vi "DatabaseHandler_Core.vi"(0 "Object Refnum In":T3, 1 "Name":string, 2 "Object Data In":T2, 3 "subele index":i32, 4 "SubEle In":T1, 5 "error in (no error)":errorcluster, 6 "Function (Get Data)":T4=enum."Get Data") -> (11 "Valid Object":bool, 12 "Objects":T3[](array[typedef]), 13 "Created New":bool, 14 "Object Refnum out":T3, 15 "Name Out":string, 16 "Object Data Out":T2, 18 "object index":i32, 19 "error out":errorcluster)   [LabVIEW 2016]
doc: "This VI is the object core. It assigns a RefNum for each object as it is created using the Register function. Object data is accessed using the appropriate RefNum.\nCopyright 2001 VI Engineering, Inc."
uses:
  Database_Refnum.ctl
  DatabaseHand_Function.ctl
  DatabaseHand_Element.ctl
  DatabaseHan_DatabaseElement.ctl
  <vilib>/Utility/error.llb/whitespace.ctl
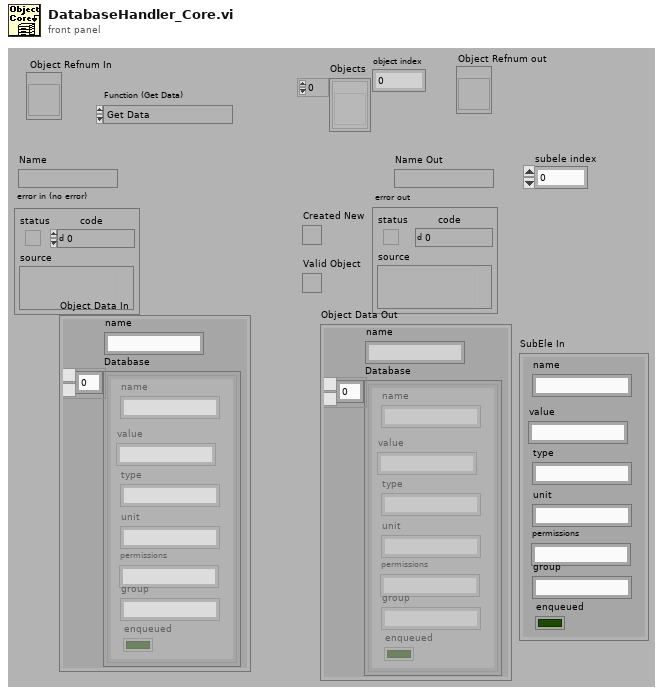
[diagram p1: front panel]
types:
  T1 = typedef "DatabaseHan_DatabaseElement.ctl" = cluster{"name":string, "value":string, "type":string, "unit":string, "permissions":string, "enqueued":bool, "group":string}
  T2 = typedef "DatabaseHand_Element.ctl" = cluster{"name":string, "Database":T1[]}
  T3 = typedef "Database_Refnum.ctl" = refnum<vi>
  T4 = typedef "DatabaseHand_Function.ctl" = enum16{"Reset", "Register", "Get Data", "Set Data", "Unregister", "Test", "Get Objects", "Delete Data"}
  T5 = typedef "whitespace.ctl" = u16
  T6 = typedef "Semaphore RefNum" = refnum<k1>
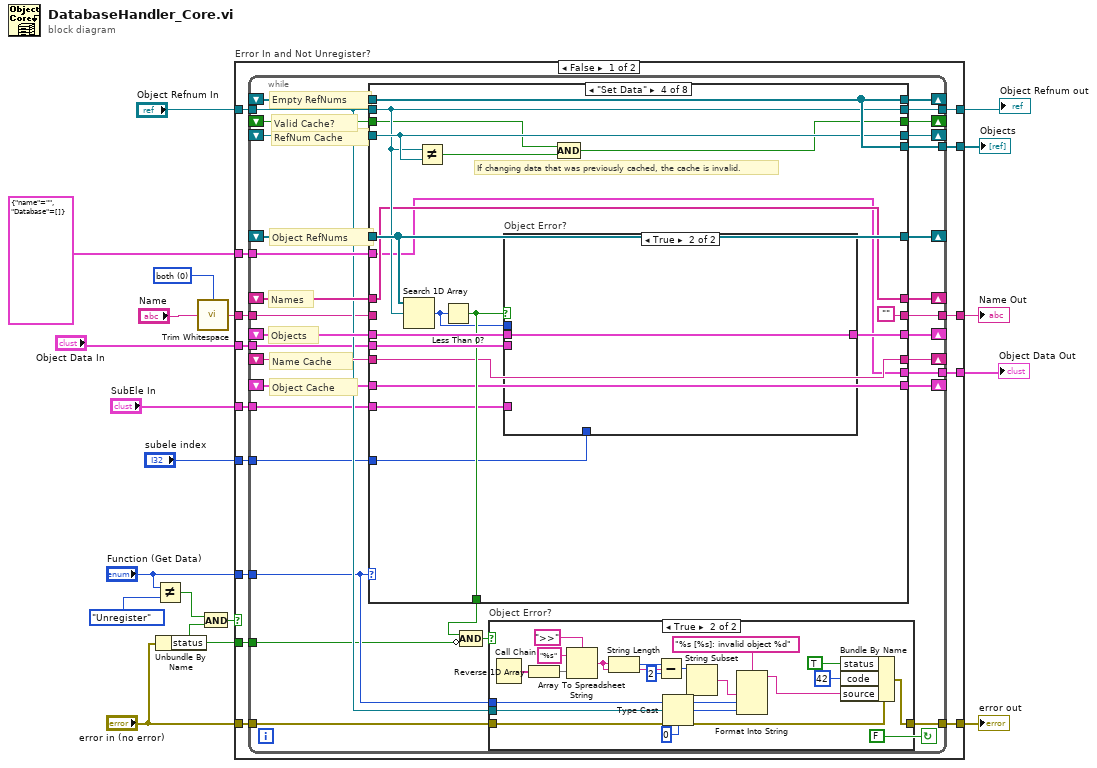
[diagram p0: block diagram]
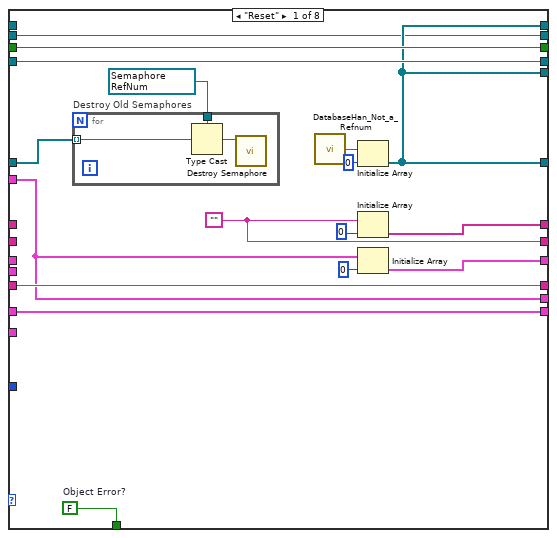
[diagram p3: hidden frame]
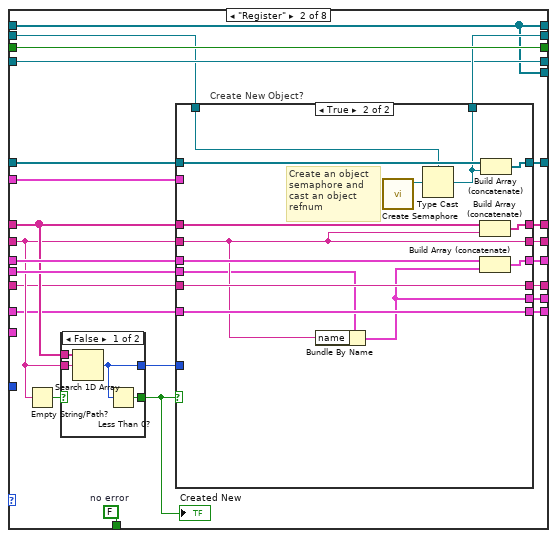
[diagram p4: hidden frame]
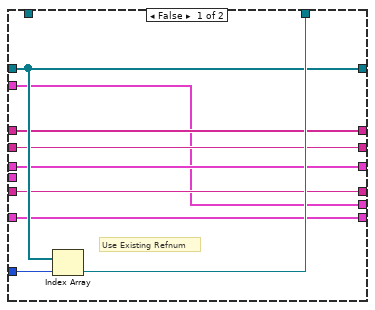
[diagram p5: hidden frame]
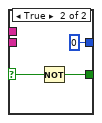
[diagram p6: hidden frame]
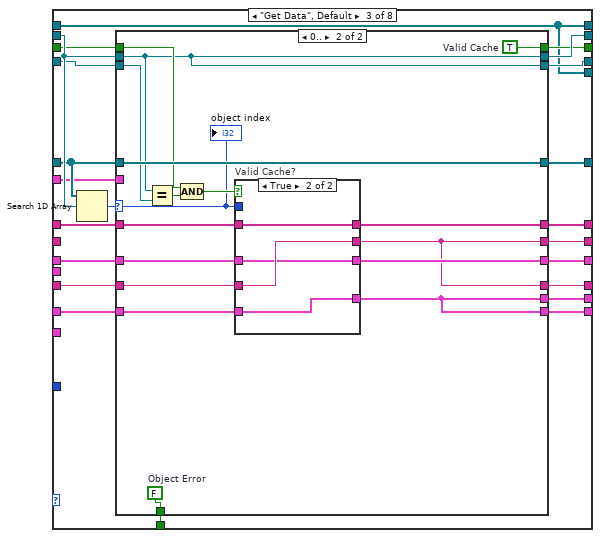
[diagram p7: hidden frame]
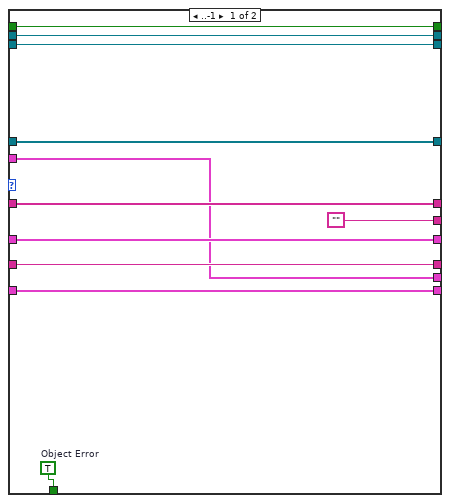
[diagram p8: hidden frame]
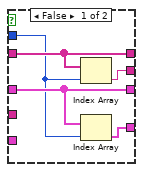
[diagram p9: hidden frame]
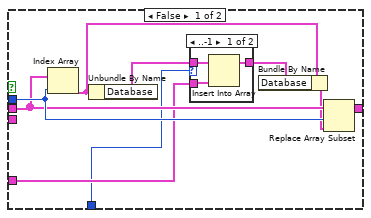
[diagram p10: hidden frame]
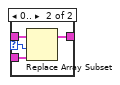
[diagram p11: hidden frame]
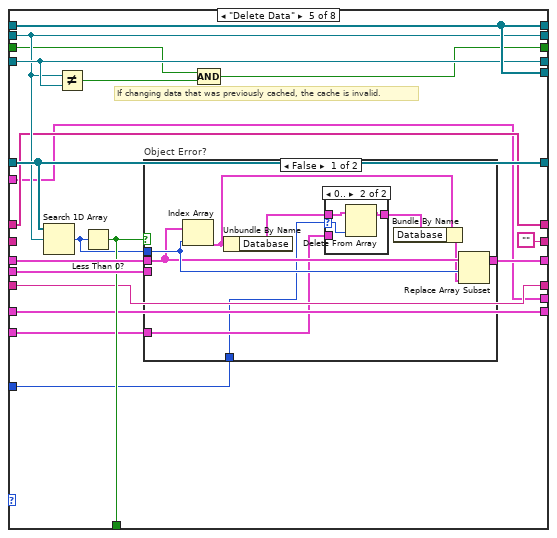
[diagram p12: hidden frame]
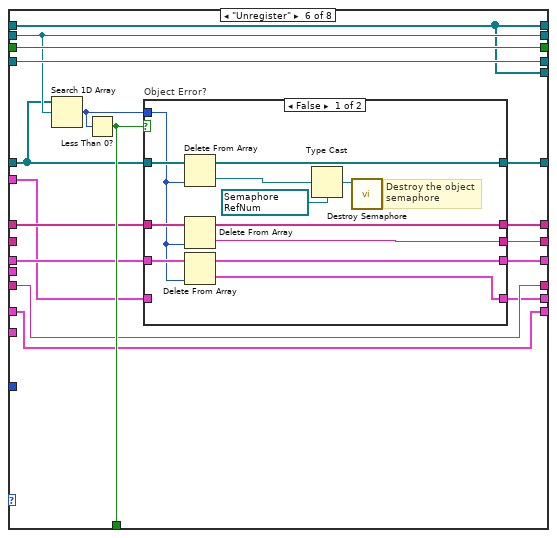
[diagram p15: hidden frame]
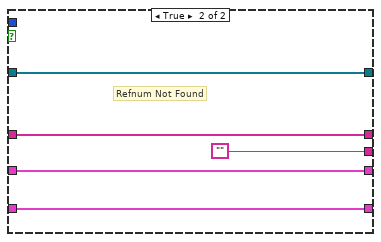
[diagram p16: hidden frame]
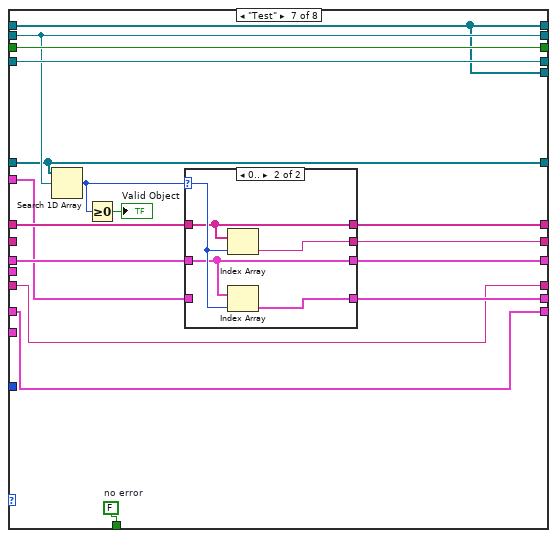
[diagram p17: hidden frame]
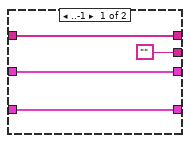
[diagram p18: hidden frame]
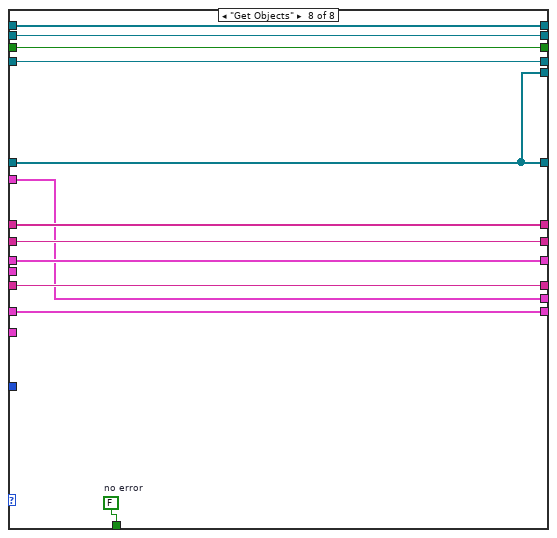
[diagram p19: hidden frame]
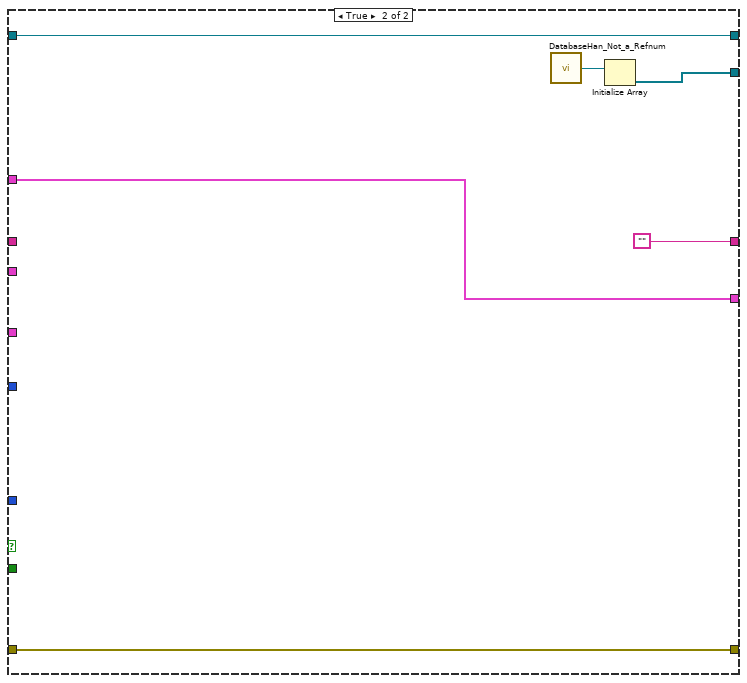
[diagram p20: hidden frame]
diagram:
  w1 = T5 0 items=["both", "start of string", "end of string"] ("location (both)")
  n1 = Not Equal?(x="Function (Get Data)", y=DatabaseHand_Function."Unregister") -> (x != y?=w13:bool)
  n2 = Unbundle By Name("error in (no error)") -> ("status"=w14:bool)
  n3 = call <vilib>:"Trim Whitespace.vi"("string"="Name", "location (both)"=w1) -> ("trimmed string"=w2:string)
  n4 = And(x=w13, y=w14) -> (x .and. y?=w12:bool)
  n5 = case "Error In and Not Unregister?" shown="False" w12 {
    tunnel: "Object Refnum In" -> [w33 w365]
    tunnel: cluster{"name":string, "Database":T1[]} {"name"="", "Database"=[]} ("Object Data In") -> [w32 w361]
    tunnel: "error in (no error)" -> [w31 w366]
    tunnel: [w30 w366] -> w19
    tunnel: "Object Data In" -> [w29 _]
    tunnel: [w28 w365] -> w10
    tunnel: w2 -> [w27 _]
    tunnel: [w26 ""] -> w17
    tunnel: [w25 w361] -> w8
    tunnel: [w24 w363] -> w6
    tunnel: "Function (Get Data)" -> [w23 _]
    tunnel: w14 -> [w22 _]
    tunnel: "SubEle In" -> [w21 _]
    tunnel: "subele index" -> [w20 _]
    frame False {
      n6 = while {
        tunnel: w22 -> [w39]
        shift-left: _ -> [w40]
        shift-right: [w41] -> _
        tunnel: [w42] -> w24
        tunnel: [w43] -> w25
        tunnel: [w44] -> w26
        tunnel: w27 -> [w45]
        tunnel: [w46] -> w28
        tunnel: w29 -> [w47]
        tunnel: [w48] -> w30
        tunnel: w31 -> [w51]
        shift-left: _ -> [w54]
        shift-right: [w53] -> _
        shift-left: _ -> [w56]
        shift-right: [w55] -> _
        shift-left: _ -> [w58]
        shift-right: [w57] -> _
        tunnel: w32 -> [w52]
        tunnel: w33 -> [w50]
        shift-left: _ -> [w60]
        shift-right: [w59] -> _
        shift-left: _ -> [w62]
        shift-right: [w61] -> _
        shift-left: _ -> [w64]
        shift-right: [w63] -> _
        shift-left: _ -> [w66]
        shift-right: [w65] -> _
        tunnel: w23 -> [w49]
        tunnel: w21 -> [w35]
        tunnel: w20 -> [w34]
        stop <- FALSE continue-if-true
        # "Empty RefNums"
        # "Object Cache"
        # "Name Cache"
        # "Names"
        # "Objects"
        # "Object RefNums"
        # "RefNum Cache"
        # "Valid Cache?"
        n7 = case shown="\"Set Data\"" w49 {
          tunnel: w50 -> [w91 w121 w181 w228 w264 w303 w337 w358]
          tunnel: w66 -> [w103 w130 w180 w225 w261 w304 w338 w359]
          tunnel: [w103 w130 w174 w227 w263 w304 w338 w359] -> w65
          tunnel: w64 -> [w102 w123 w179 w229 w265 w305 w339 w360]
          tunnel: [w102 w123 w173 w229 w265 w305 w339 w360] -> w63
          tunnel: w62 -> [w87 w122 w178 w231 w267 w301 w336 w349]
          tunnel: [w92 w129 w172 w231 w267 w298 w336 w349] -> w61
          tunnel: w60 -> [_ w128 w177 w237 w273 w299 w332 w352]
          tunnel: [w98 w127 w171 w236 w272 w295 w328 w352] -> w59
          tunnel: w58 -> [_ w120 w176 w226 w262 w300 w333 w354]
          tunnel: [w93 w124 w170 w226 w262 w296 w329 w354] -> w57
          tunnel: w56 -> [w101 w116 w169 w233 w269 w294 w325 w355]
          tunnel: [w101 w115 w165 w233 w269 w294 w325 w355] -> w55
          tunnel: w54 -> [w100 w114 w168 w232 w268 w293 w326 w356]
          tunnel: [w100 w113 w164 w232 w268 w293 w326 w356] -> w53
          tunnel: w52 -> [w89 w110 w162 w222 w258 w289 w327 w351]
          tunnel: [w95 w108 w163 w235 w271 w302 w335 w357] -> w37
          tunnel: w47 -> [_ w126 _ w238 w274 _ _ _]
          tunnel: [w91 w125 w175 w228 w264 w303 w337 w358] -> w46
          tunnel: w45 -> [_ w119 _ _ _ _ _ w353]
          tunnel: [w90 w112 w167 "" "" w291 w331 w353] -> w44
          tunnel: [w89 w111 w166 w222 w258 w290 w330 w351] -> w43
          tunnel: [w92 w109 w161 w230 w266 w292 w324 w349] -> w42
          tunnel: [w92 w109 w161 w230 w266 w292 w324 w350] -> w41
          tunnel: w40 -> [_ w109 w161 w230 w266 w292 w324 w350]
          tunnel: w35 -> [_ _ _ w221 w257 _ _ _]
          tunnel: w34 -> [_ _ _ w220 w256 _ _ _]
          frame "Reset" {
            w88 = T6 refnum items=["semaphore"] ("semaphore")
            w95 = FALSE  # Object Error?
            w90 = ""
            n8 = for "Destroy Old Semaphores" {
              tunnel: w87 -> [w105] mode=indexing
              tunnel: w88 -> [w106]
              n9 = Type Cast(type=w106, x=w105) -> (*(type *) &x=w104:T6)
              n10 = call <vilib>:"Destroy Semaphore.vi"("semaphore"=w104) -> ()  [unwired: 1 in, 6 out]
            }
            n11 = call "DatabaseHan_Not_a_Refnum.vi"() -> ("Not_an_element_Refnum"=w96:T3)
            n12 = Initialize Array(w96, 0 ("Dimension Size")) -> (w92:T3[])
            n13 = Initialize Array(w90, 0 ("Dimension Size")) -> (w93:string[])
            n14 = Initialize Array(w89, 0 ("Dimension Size")) -> (w98:cluster{"name":string, "Database":T1[]}[])
          }
          frame "Register" {
            w108 = FALSE  # no error
            n15 = Empty String/Path?(string/path=w119) -> (empty?=w118:bool)
            n16 = case shown="False" w118 {
              selector: w118 -> [_ w160]
              tunnel: w120 -> [w157 _]
              tunnel: w119 -> [w156 _]
              tunnel: [w155 0 ("index of element")] -> w117
              tunnel: [w154 w158] -> w107
              frame False {
                n17 = Search 1D Array(1D array=w157, element=w156) -> (index of element=w155:i32)  [unwired: 1 out]
                n18 = Less Than 0?(x=w155) -> (x < 0?=w154:bool)
              }
              frame True {
                n19 = Not(x=w160) -> (.not. x?=w158:bool)
              }
            }
            "Created New" <- w107
            n20 = case "Create New Object?" shown="True" w107 {
              tunnel: [w138 w153] -> w129
              tunnel: w128 -> [w135 w152]
              tunnel: [w135 w151] -> w127
              tunnel: w126 -> [_ w141]
              tunnel: [w139 w143] -> w125
              tunnel: [w137 w150] -> w124
              tunnel: w122 -> [w138 w149]
              tunnel: w121 -> [_ w144]
              tunnel: w120 -> [w137 w148]
              tunnel: w119 -> [w136 w142]
              tunnel: w117 -> [w131 _]
              tunnel: w116 -> [w134 w147]
              tunnel: [w134 w147] -> w115
              tunnel: w114 -> [w133 w146]
              tunnel: [w133 w146] -> w113
              tunnel: [w136 w142] -> w112
              tunnel: [w132 w140] -> w111
              tunnel: w110 -> [w132 _]
              frame False {
                # "Use Existing Refnum"
                n21 = Index Array(array=w138, index=w131) -> (element=w139:T3)
              }
              frame True {
                # "Create an object semaphore and cast an object refnum"
                n22 = Bundle By Name(cluster=w141, "name"=w142) -> (w140:T2)
                n23 = call <vilib>:"Create Semaphore.vi"() -> ("semaphore"=w145:T6)  [unwired: 2 in, 5 out]
                n24 = Type Cast(type=w144, x=w145) -> (*(type *) &x=w143:T3)
                n25 = Build Array (concatenate)(w148, w142) -> (w150:string[])
                n26 = Build Array (concatenate)(w152, w140) -> (w151:T2[])
                n27 = Build Array (concatenate)(w149, w143) -> (w153:T3[])
              }
            }
          }
          frame "Get Data", Default {
            n28 = Search 1D Array(1D array=w178, element=w181) -> (index of element=w182:i32)  [unwired: 1 out]
            n29 = case shown="0.." w182 {
              selector: w182 -> [_ w194]
              tunnel: w181 -> [w189 w199]
              tunnel: w180 -> [w188 w200]
              tunnel: w179 -> [w187 w208]
              tunnel: w178 -> [w186 w210]
              tunnel: w177 -> [w192 w204]
              tunnel: w176 -> [w193 w203]
              tunnel: [w189 w199] -> w175
              tunnel: [w188 w198] -> w174
              tunnel: [w187 w199] -> w173
              tunnel: [w186 w210] -> w172
              tunnel: [w192 w202] -> w171
              tunnel: [w193 w201] -> w170
              tunnel: w169 -> [w190 w206]
              tunnel: w168 -> [w191 w205]
              tunnel: ["" w197] -> w167
              tunnel: [w184 w196] -> w166
              tunnel: [w190 w197] -> w165
              tunnel: [w191 w196] -> w164
              tunnel: [w185 w195] -> w163
              tunnel: w162 -> [w184 _]
              frame ..-1 {
                w185 = TRUE  # Object Error
              }
              frame 0.. {
                w195 = FALSE  # Object Error
                w198 = TRUE  # Valid Cache
                n30 = Equal?(x=w199, y=w208) -> (x = y?=w209:bool)
                n31 = Compound Arithmetic op=AND(w200, w209) -> (w207:bool)
                n32 = case "Valid Cache?" shown="True" w207 {
                  tunnel: w206 -> [_ w219]
                  tunnel: w205 -> [_ w218]
                  tunnel: w204 -> [w213 w217]
                  tunnel: w203 -> [w212 w216]
                  tunnel: [w215 w219] -> w197
                  tunnel: [w214 w218] -> w196
                  tunnel: w194 -> [w211 _]
                  tunnel: [w213 w217] -> w202
                  tunnel: [w212 w216] -> w201
                  frame False {
                    n33 = Index Array(array=w212, index=w211) -> (element=w215:string)
                    n34 = Index Array(array=w213, index=w211) -> (element=w214:T2)
                  }
                  frame True {
                  }
                }
                "object index" <- w194
              }
            }
          }
          frame "Set Data" {
            # "If changing data that was previously cached, the cache is invalid."
            n35 = Search 1D Array(1D array=w231, element=w228) -> (index of element=w223:i32)  [unwired: 1 out]
            n36 = Not Equal?(x=w228, y=w229) -> (x != y?=w224:bool)
            n37 = Less Than 0?(x=w223) -> (x < 0?=w235:bool)
            n38 = case "Object Error?" shown="True" w235 {
              tunnel: w238 -> [_ _]
              tunnel: w237 -> [w245 w255]
              tunnel: [w247 w255] -> w236
              tunnel: w223 -> [w246 _]
              tunnel: w221 -> [w240 _]
              tunnel: w220 -> [w239 _]
              frame False {
                n39 = Index Array(array=w245, index=w246) -> (element=w242:T2)
                n40 = Unbundle By Name(w242) -> ("Database"=w244:T1[])
                n41 = case shown="..-1" w239 {
                  selector: w239 -> [_ w251]
                  tunnel: w244 -> [w248 w254]
                  tunnel: w240 -> [w250 w253]
                  tunnel: [w249 w252] -> w243
                  frame ..-1 {
                    n42 = Insert Into Array(array=w248, new element=w250) -> (w249:T1[])  [unwired: 1 in]
                  }
                  frame 0.. {
                    n43 = Replace Array Subset(array=w254, new element=w253, index=w251) -> (w252:T1[])
                  }
                }
                n44 = Bundle By Name(cluster=w242, "Database"=w243) -> (w241:T2)
                n45 = Replace Array Subset(array=w245, new element=w241, index=w246) -> (w247:T2[])
              }
              frame True {
              }
            }
            n46 = Compound Arithmetic op=AND(w225, w224) -> (w227:bool)
          }
          frame "Delete Data" {
            # "If changing data that was previously cached, the cache is invalid."
            n47 = Search 1D Array(1D array=w267, element=w264) -> (index of element=w259:i32)  [unwired: 1 out]
            n48 = Not Equal?(x=w264, y=w265) -> (x != y?=w260:bool)
            n49 = Less Than 0?(x=w259) -> (x < 0?=w271:bool)
            n50 = case "Object Error?" shown="False" w271 {
              tunnel: w274 -> [_ _]
              tunnel: w273 -> [w281 w288]
              tunnel: [w283 w288] -> w272
              tunnel: w259 -> [w282 _]
              tunnel: w257 -> [w276 _]
              tunnel: w256 -> [w275 _]
              frame False {
                n51 = Index Array(array=w281, index=w282) -> (element=w278:T2)
                n52 = Unbundle By Name(w278) -> ("Database"=w280:T1[])
                n53 = case shown="0.." w275 {
                  selector: w275 -> [_ w285]
                  tunnel: w280 -> [w284 w287]
                  tunnel: w276 -> [_ _]
                  tunnel: [w284 w286] -> w279
                  frame ..-1 {
                  }
                  frame 0.. {
                    n54 = Delete From Array(array=w287, index=w285) -> (array with subset deleted=w286:T1[])  [unwired: 1 in, 1 out]
                  }
                }
                n55 = Bundle By Name(cluster=w278, "Database"=w279) -> (w277:T2)
                n56 = Replace Array Subset(array=w281, new element=w277, index=w282) -> (w283:T2[])
              }
              frame True {
              }
            }
            n57 = Compound Arithmetic op=AND(w261, w260) -> (w263:bool)
          }
          frame "Unregister" {
            n58 = Search 1D Array(1D array=w301, element=w303) -> (index of element=w297:i32)  [unwired: 1 out]
            n59 = Less Than 0?(x=w297) -> (x < 0?=w302:bool)
            n60 = case "Object Error?" shown="False" w302 {
              tunnel: w301 -> [w317 w320]
              tunnel: w300 -> [w315 w322]
              tunnel: w299 -> [w313 w321]
              tunnel: [w316 w320] -> w298
              tunnel: w297 -> [w309 _]
              tunnel: [w314 w322] -> w296
              tunnel: [w312 w321] -> w295
              tunnel: [w311 ""] -> w291
              tunnel: [w310 w318] -> w290
              tunnel: w289 -> [_ w318]
              frame False {
                w308 = T6 refnum items=["semaphore"] ("semaphore")
                # "Destroy the object semaphore"
                n61 = Delete From Array(array=w317, index=w309) -> (deleted portion=w307:T3, array with subset deleted=w316:T3[])  [unwired: 1 in]
                n62 = Delete From Array(array=w315, index=w309) -> (deleted portion=w311:string, array with subset deleted=w314:string[])  [unwired: 1 in]
                n63 = Delete From Array(array=w313, index=w309) -> (deleted portion=w310:T2, array with subset deleted=w312:T2[])  [unwired: 1 in]
                n64 = Type Cast(type=w308, x=w307) -> (*(type *) &x=w306:T6)
                n65 = call <vilib>:"Destroy Semaphore.vi"("semaphore"=w306) -> ()  [unwired: 1 in, 6 out]
              }
              frame True {
                # "Refnum Not Found"
              }
            }
          }
          frame "Test" {
            w335 = FALSE  # no error
            n66 = Search 1D Array(1D array=w336, element=w337) -> (index of element=w323:i32)  [unwired: 1 out]
            n67 = Greater Or Equal To 0?(x=w323) -> (x >= 0?=→"Valid Object":bool)
            n68 = case shown="0.." w323 {
              selector: w323 -> [_ w348]
              tunnel: w333 -> [w343 w345]
              tunnel: w332 -> [w342 w344]
              tunnel: ["" w347] -> w331
              tunnel: [w340 w346] -> w330
              tunnel: [w343 w345] -> w329
              tunnel: [w342 w344] -> w328
              tunnel: w327 -> [w340 _]
              frame ..-1 {
              }
              frame 0.. {
                n69 = Index Array(array=w345, index=w348) -> (element=w347:string)
                n70 = Index Array(array=w344, index=w348) -> (element=w346:T2)
              }
            }
          }
          frame "Get Objects" {
            w357 = FALSE  # no error
          }
        }
        n71 = Compound Arithmetic op=AND(w37, invert w39) -> (w38:bool)
        n72 = case "Object Error?" shown="True" w38 {
          tunnel: w49 -> [_ w84]
          tunnel: w50 -> [_ w85]
          tunnel: w51 -> [w67 w80]
          tunnel: [w67 w81] -> w48
          frame False {
          }
          frame True {
            n73 = Call Chain() -> (call chain=w79:string[])
            n74 = Reverse 1D Array(array=w79) -> (reversed array=w77:string[])
            n75 = Array To Spreadsheet String(delimiter (Tab)=">>", array=w77, 3:"%s" ("format string")) -> (spreadsheet string=w72:string)
            n76 = String Length(string=w72) -> (length=w75:i32)
            n77 = Subtract(x=w75, y=2) -> (x-y=w73:i32)
            n78 = Type Cast(type=u32 0 ("object"), x=w85) -> (*(type *) &x=w83:u32)
            n79 = String Subset(string=w72, length (rest)=w73) -> (substring=w71:string)  [unwired: 1 out]
            n80 = Format Into String(format string="%s [%s]: invalid object %d", w71, w84, w83) -> (resulting string=w70:string)  [unwired: 2 in, 1 out]
            n81 = Bundle By Name(cluster=w80, "status"=TRUE ("Bundle Element"), "code"=42 ("Bundle Element"), "source"=w70) -> (w81:errorcluster)
          }
        }
      }
    }
    frame True {
      n82 = call "DatabaseHan_Not_a_Refnum.vi"() -> ("Not_an_element_Refnum"=w364:T3)
      n83 = Initialize Array(w364) -> (w363:T3[])  [unwired: 1 out]
    }
  }
  "Objects" <- w6
  "error out" <- w19
  "Name Out" <- w17
  "Object Refnum out" <- w10
  "Object Data Out" <- w8
